vi "N Field Set Com.vi"(2 "command text in":string[](array[string]), 3 "option":T2) -> (1 "Command text out":string[][](array[string]))   [LabVIEW 2020]
uses:
  Ctl/option.ctl
  Field Set.ctl
panel:
  in  "SetFieldCluster":T1={"rate"=0.0005, "set point"=0.0, "extra wait"=5, "wait option"=1} {"wait option" items=["Do not wait, just move on", "Wait until it reaches the set point."]; "extra wait" min=0; "set point" format="%.5f"; "rate" format="%.5f"}
  in  "enter":bool
  in  "cancel":bool
  # "Set Field Command"
  # "T"
  # "at"
  # "T/min"
  # "1. Sweep field to"
  # "2. AND wait extra"
  # "seconds"
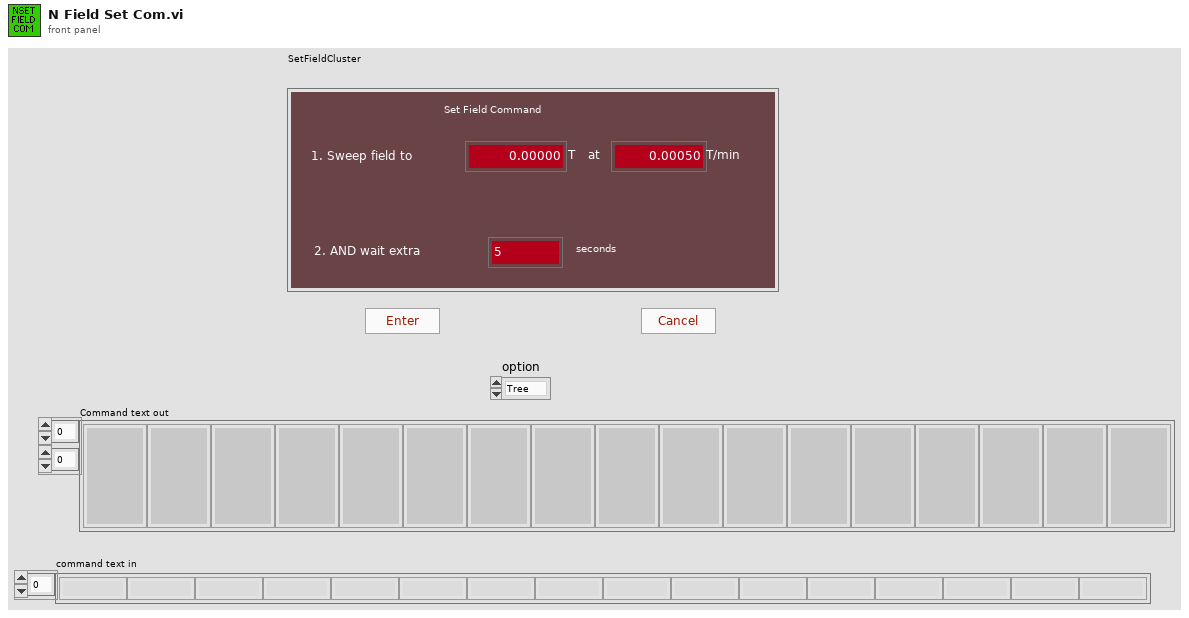
[diagram p1: front panel]
types:
  T1 = typedef "Field Set.ctl" = cluster{"rate":dbl, "set point":dbl, "extra wait":i32, "wait option":u16}
  T2 = typedef "option.ctl" = enum16{"Tree", "List"}
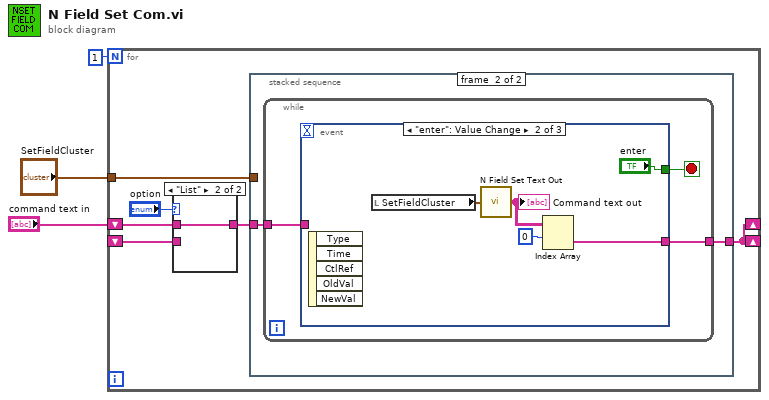
[diagram p0: block diagram]
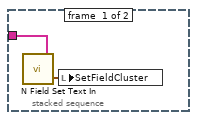
[diagram p3: hidden frame]
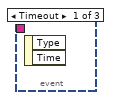
[diagram p4: hidden frame]
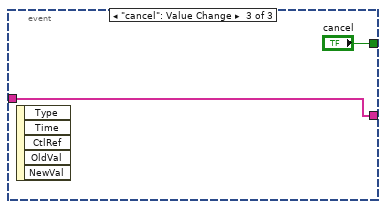
[diagram p5: hidden frame]
diagram:
  n1 = for {
    N: 1 -> [_]
    shift-right: [w6] -> _
    shift-left: _ -> [w8]
    shift-right: [w6] -> _
    shift-left: "command text in" -> [w7]
    tunnel: "SetFieldCluster" -> [w4]
    n2 = case shown="\"List\"" "option" {
      tunnel: [w10 w11] -> w9
      tunnel: w8 -> [w10 _]
      tunnel: w7 -> [_ w11]
      frame "Tree", Default {
      }
      frame "List" {
      }
    }
    n3 = stacked-sequence {
      tunnel: [_ w15] -> w6
      tunnel: w9 -> [w13 w14]
      tunnel: w4 -> [_ _]
      frame #0 {
        n4 = call "N Field Set Text In.vi"("command text in"=w13) -> ("SetFieldCluster"=w12:T1)  [unwired: 4 in]
        n5 = local write "SetFieldCluster"(w12) -> ()
      }
      frame #1 {
        n6 = while {
          tunnel: [w17] -> w15
          tunnel: w14 -> [w16]
          stop <- w18 stop-if-true
          n7 = event shown="[1] \"enter\": Value Change" {
            selector: _ -> [_ _ _]
            dyn-events: _ -> [_ _ _]
            timeout: _ -> [_ _ _]
            tunnel: [_ "enter" "cancel"] -> w18
            tunnel: [_ w20 w24] -> w17
            tunnel: w16 -> [_ _ w24]
            event Timeout {
              n8 = event-data() -> ()  [unwired: 1 in, 2 out]
            }
            event "enter": Value Change {
              n9 = event-data() -> ()  [unwired: 1 in, 5 out]
              n10 = local read "SetFieldCluster"() -> (w19:T1)
              n11 = call "N Field Set Text Out.vi"("SetFieldCluster"=w19) -> ("Command text"=w22:string[][])
              "Command text out" <- w22
              n12 = Index Array(array=w22, index (row)=0) -> (element=w20:string[])  [unwired: 1 in]
            }
            event "cancel": Value Change {
              n13 = event-data() -> ()  [unwired: 1 in, 5 out]
            }
          }
        }
      }
    }
  }
